vi "Wrist Controller.vi"(8 "error in":errorcluster) -> ()   [LabVIEW 2018]
doc: "This VI executes continuously carrying out the current operation and responding to updates or new operations. It will often contain the timing or control code that is difficult to place directly in TeleOp. This VI generally opens all sensors and motors and isolates the rest of the robot code from knowing how the operations are carried out."
uses:
  <vilib>/Rock Robotics/WPI/Framework/Completion Status.ctl
  Wrist Setpoints.ctl
  Wrist Operations.ctl
  <vilib>/Rock Robotics/WPI/MotorControl/WPI_MotorControlDeviceRef.ctl
  <vilib>/Rock Robotics/WPI/MotorControl/WPI_MotorControlType.ctl
  <vilib>/Rock Robotics/SystemInterfaces/DIO/FPGA_DIOPWMChannel.ctl
  <vilib>/Rock Robotics/WPI/PWM/WPI_PWMDeadband.ctl
  <vilib>/Rock Robotics/SystemInterfaces/DIO/FPGA_DIOChannel.ctl
  <vilib>/Rock Robotics/WPI/Counter/WPI_CounterDevRef.ctl
  <vilib>/Rock Robotics/SystemInterfaces/Counter/FPGA_CounterCtrSystemIndex.ctl
  <vilib>/Rock Robotics/WPI/ThirdParty/REV Robotics/SPARK MAX/Typedef/Spark MAX Control Type.ctl
  Wrist Published Globals.vi
panel:
  in  "Sensor Distance":dbl=190.0
  in  "0 Offset":dbl=160.0
  in  "Gravity Voltage":dbl=-0.5
  in  "upper limit":dbl=107.0
  in  "lower limit":dbl=-10.0
  in  "invert?":bool=TRUE
  in  "i Zone":dbl=inf format="%.2f"
  in  "PIDF gains":cluster{"Kp":dbl, "Ki":dbl, "Kd":dbl, "Kf":dbl}={"Kp"=0.03, "Ki"=0.0, "Kd"=0.0, "Kf"=0.0} {"Kf" format="%.3f"; "Kd" format="%.3f"; "Ki" format="%.3f"; "Kp" format="%.3f"}
  in  "output range":cluster{"output high":dbl, "output low":dbl}={"output high"=0.75, "output low"=-0.75} {"output low" format="%.2f"; "output high" format="%.2f"}
  out "Waveform Chart":T1(graph)={"output"=-0.11472656249999999, "upper limit"=105.0, "unwrapped phase"=101.17578125}
  in  "Interactive Values":T2={"Operation"=enum."Set Position", "Setpoint"=50.0, "Duration"=0.0}
  out "Current\nCmd":string="Started at  19:12:07.827\nDefault: Reserve,  S 0.0, D 0.000000"
  in  "Buttons":cluster{"Execute Cmd":bool, "Abort Cmd":bool}
  out "Command Timing":cluster{"Start Time (ms)":u32, "Iterations":i32}={"Start Time (ms)"=1785240, "Iterations"=0}
  out "Status":T4
  # "Interactive Command: You may fill in the settings for a command\nand schedule it with the Execute button. You can observe and abort\nany command while fine tuning the code for the controller."
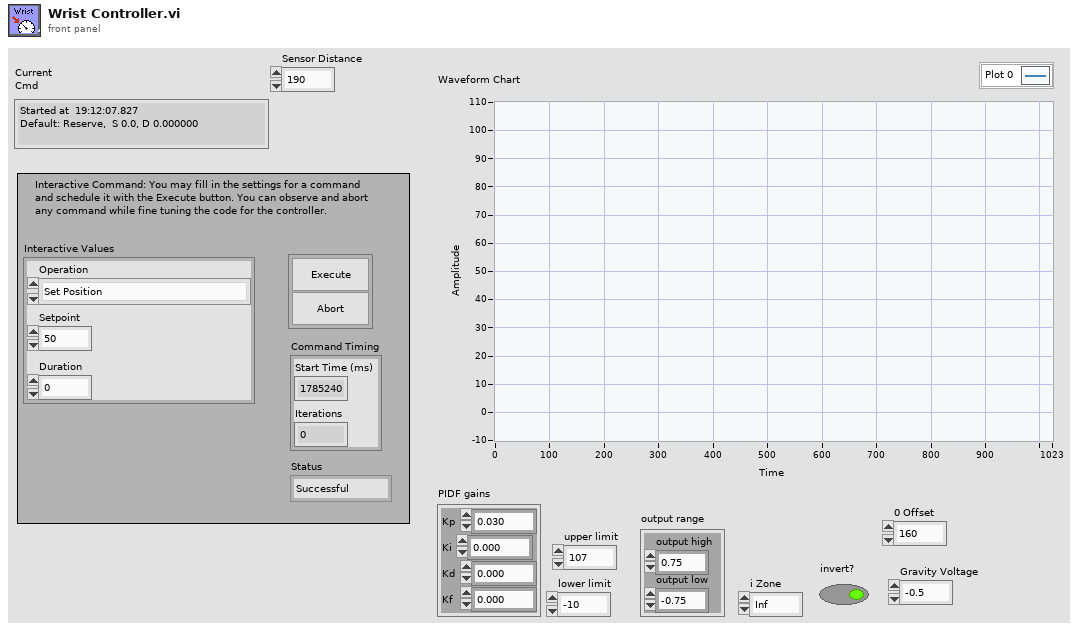
[diagram p1: front panel]
types:
  T1 = cluster{"output":dbl, "upper limit":dbl, "unwrapped phase":dbl}
  T2 = typedef "Wrist Setpoints.ctl" = cluster{"Operation":T3, "Setpoint":dbl, "Duration":dbl}
  T3 = typedef "Wrist Operations.ctl" = enum16{"Reserve", "Read Current", "Immediate", "Set Position"}
  T4 = typedef "Completion Status.ctl" = enum16{"Successful", "Aborted", "Incomplete"}
  T5 = typedef "WPI_MotorControlDeviceRef.ctl" = cluster{"DeviceStatus":errorcluster, "Type":T6, "PWM":cluster{"PWM Channel":T7, "DeadBand":T8}, "CAN":cluster{"Device Number":u8, "SetOutput VI Ref":variant, "GetOutput VI Ref":variant, "Enable VI Ref":variant, "Disable VI Ref":variant, "Data":variant}, "Invert":bool, "DIO PWM":cluster{"PWM \"Enable\" Channel":T7, "DIOChannel":T9, "PWM Rate":dbl}}
  T6 = typedef "WPI_MotorControlType.ctl" = enum16{"PWM", "CAN", "DIO PWM"}
  T7 = typedef "FPGA_DIOPWMChannel.ctl" = enum8{"PWM 0", "PWM 1", "PWM 2", "PWM 3", "PWM 4", "PWM 5", "PWM 6", "PWM 7", "PWM 8", "PWM 9", "PWM MXP 0", "PWM MXP 1", "PWM MXP 2", "PWM MXP 3", "PWM MXP 4", "PWM MXP 5", "PWM MXP 6", "PWM MXP 7", "PWM MXP 8", "PWM MXP 9", "Invalid"}
  T8 = typedef "WPI_PWMDeadband.ctl" = cluster{"Name":string, "maxPositivePwm":i32, "minPositivePwm":i32, "centerPwm":i32, "maxNegativePwm":i32, "minNegativePwm":i32, "angularRange":u16}
  T9 = typedef "FPGA_DIOChannel.ctl" = enum8{"DIO 0", "DIO 1", "DIO 2", "DIO 3", "DIO 4", "DIO 5", "DIO 6", "DIO 7", "DIO 8", "DIO 9", "DIO MXP 0", "DIO MXP 1", "DIO MXP 2", "DIO MXP 3", "DIO MXP 4", "DIO MXP 5", "DIO MXP 6", "DIO MXP 7", "DIO MXP 8", "DIO MXP 9", "DIO MXP 10", "DIO MXP 11", "DIO MXP 12", "DIO MXP 13", "DIO MXP 14", "DIO MXP 15", "SPI Port CS1", "SPI Port CS2", "SPI Port CS3", "SPI Port MISO", "SPI Port MOSI", "Invalid"}
  T10 = typedef "WPI_CounterDevRef.ctl" = cluster{"DevStatus":errorcluster, "CntIndex":T11}
  T11 = typedef "FPGA_CounterCtrSystemIndex.ctl" = enum8{"Ctr 0", "Ctr 1", "Ctr 2", "Ctr 3", "Ctr 4", "Ctr 5", "Ctr 6", "Ctr 7", "Invalid"}
  T12 = cluster{"Motor":T5, "Sensor":T10, "Setpoint":dbl, "Cargo Detect":T10}
  T13 = typedef "Command Status Info.ctl" = cluster{"Name":string, "Status":T4, "notifier out":T14}
  T14 = typedef "Completion Notifier.ctl" = refnum<notifier>
  T15 = cluster{"Current Command":T2, "Command Timing":cluster{"Start Time (ms)":u32, "Iterations":i32}, "Command Arguments":cluster{"Command Info":T13, "Description":string, "Default Command":T2, "queue out":refnum<queue>, "Subsystem Name":string}}
  T16 = typedef "Spark MAX Control Type.ctl" = enum16{"Percent VBus", "Voltage", "Velocity", "Position", "Smart Motion", "Current", "Smart Velocity"}
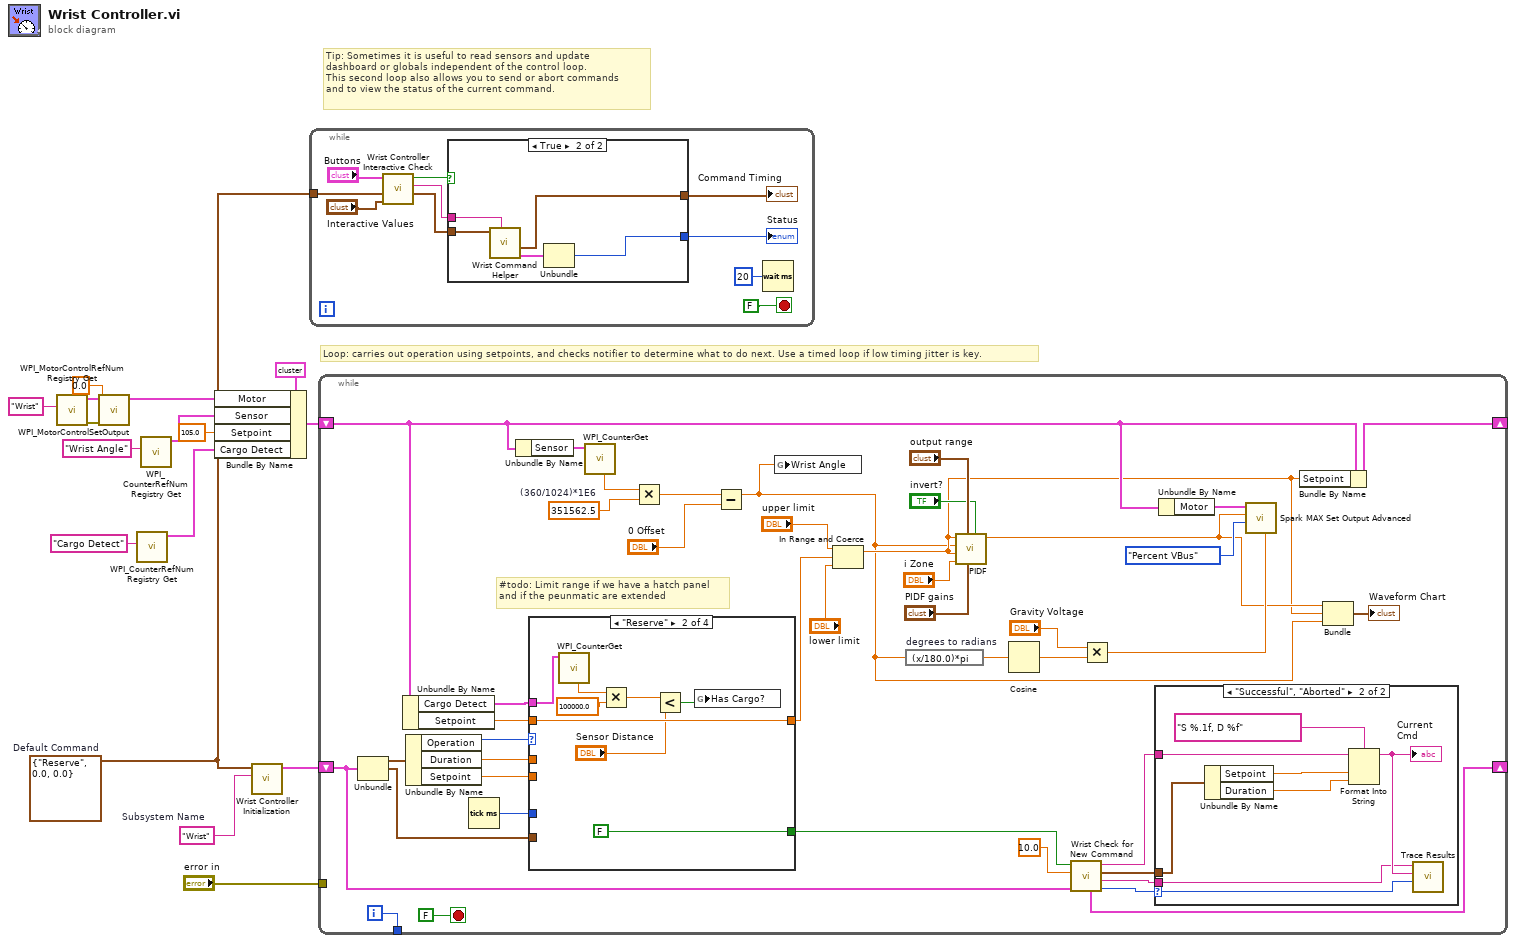
[diagram p0: block diagram]
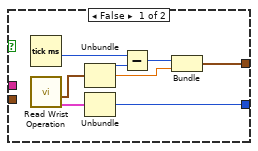
[diagram p2: hidden frame]
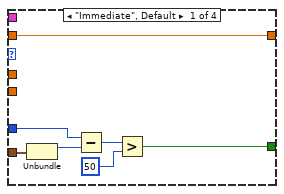
[diagram p4: hidden frame]
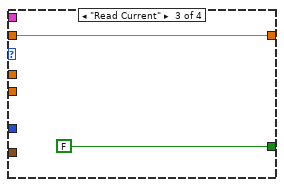
[diagram p5: hidden frame]
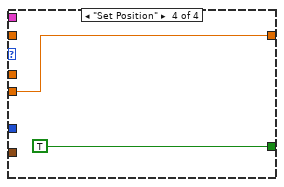
[diagram p6: hidden frame]
diagram:
  w13 = T2 {"Operation"=enum."Reserve", "Setpoint"=0.0, "Duration"=0.0}  # Default Command
  w14 = "Wrist"  # Subsystem Name
  # "Tip: Sometimes it is useful to read sensors and update\ndashboard or globals independent of the control loop.\nThis second loop also allows you to send or abort commands\nand to view the status of the current command."
  # "Loop: carries out operation using setpoints, and checks notifier to determine what to do next. Use a timed loop if low timing jitter is key."
  n1 = call <vilib>:"WPI_MotorControlRefNum Registry Get.vi"("refnum name"="Wrist") -> ("error out"=w5:errorcluster, "MotorControlDevRef"=w6:T5)  [unwired: 9 in]
  n2 = call <vilib>:"WPI_MotorControlSetOutput.vi"("error in (no error)"=w5, "Output"=0.0, "MotorControlDevRef"=w6) -> ("MotorControlDevRef"=w4:T5)  [unwired: 6 in, 2 out]
  n3 = call <vilib>:"WPI_CounterRefNum Registry Get.vi"("refnum name"="Cargo Detect") -> ("CounterDevRef"=w1:T10)  [unwired: 9 in, 1 out]
  n4 = call <vilib>:"WPI_CounterRefNum Registry Get.vi"("refnum name"="Wrist Angle") -> ("CounterDevRef"=w8:T10)  [unwired: 9 in, 1 out]
  n5 = Bundle By Name(cluster=T12 {"Motor"={"DeviceStatus"={"status"=FALSE, "code"=0, "source"=""}, "Type"=enum."PWM", "PWM"={"PWM Channel"=enum."Invalid", "DeadBand"={"Name"="", "maxPositivePwm"=0, "minPositivePwm"=0, "centerPwm"=0, "maxNegativePwm"=0, "minNegativePwm"=0, "angularRange"=0}}, "CAN"={"Device Number"=0, "SetOutput VI Ref"=variant(refnum<vi> refnum), "GetOutput VI Ref"=variant(refnum<vi> refnum), "Enable VI Ref"=variant(refnum<vi> refnum), "Disable VI Ref"=variant(refnum<vi> refnum), "Data"=variant}, "Invert"=FALSE, "DIO PWM"={"PWM \"Enable\" Channel"=enum."Invalid", "DIOChannel"=enum."Invalid", "PWM Rate"=0.0}}, "Sensor"={"DevStatus"={"status"=FALSE, "code"=0, "source"=""}, "CntIndex"=enum."Ctr 0"}, "Setpoint"=0.0, "Cargo Detect"={"DevStatus"={"status"=FALSE, "code"=0, "source"=""}, "CntIndex"=enum."Ctr 0"}}, "Motor"=w4, "Sensor"=w8, "Setpoint"=105.0, "Cargo Detect"=w1) -> (w9:T12)
  n6 = call "Wrist Controller Initialization.vi"("Subsystem Name"=w14, "Default Command"=w13) -> ("Current Command"=w15:T15)  [unwired: 9 in]
  n7 = while {
    tunnel: w13 -> [w23]
    stop <- FALSE stop-if-true
    n8 = call "Wrist Controller Interactive Check.vi"("Interactive Command in"="Interactive Values", "Default Command"=w23, "Buttons"="Buttons") -> ("Interactive Command out"=w20:T2, "Trace String"=w21:string, "Schedule"=w22:bool)  [unwired: 6 in]
    n9 = case shown="True" w22 {
      tunnel: [w34 w39] -> w19
      tunnel: w20 -> [_ w37]
      tunnel: [w30 w35] -> w18
      tunnel: w21 -> [_ w38]
      frame False {
        n10 = Tick Count (ms)() -> (millisecond timer value=w29:u32)
        n11 = call "Read Wrist Operation.vi"() -> ("Command Info"=w27:T13, "SubSystem Data"=w28:T2)  [unwired: 9 in, 1 out]
        n12 = Unbundle(w28) -> ("Operation"=w33:T3, "Setpoint"=w31:dbl)  [unwired: 1 out]
        n13 = Unbundle(w27) -> ("Status"=w34:T4)  [unwired: 2 out]
        n14 = Subtract(x=w29, y=w33) -> (x-y=w32:u32)
        n15 = Bundle(w32, "Setpoint"=w31) -> (w30:cluster{u32, "Setpoint":dbl})  [unwired: 1 in]
      }
      frame True {
        n16 = call "Wrist Command Helper.vi"("Description"=w38, "SubSystem Data"=w37) -> ("Command Info Out"=w36:T13, "Command Timing"=w35:cluster{"Start Time (ms)":u32, "Iterations":i32})  [unwired: 7 in, 1 out]
        n17 = Unbundle(w36) -> ("Status"=w39:T4)  [unwired: 2 out]
      }
    }
    "Status" <- w19
    "Command Timing" <- w18
    n18 = Wait (ms)(milliseconds to wait=u32 20) -> ()  [unwired: 1 out]
  }
  n19 = while {
    shift-right: [w73] -> _
    shift-left: w15 -> [w67]
    tunnel: [w80] -> _
    tunnel: "error in" -> [_]
    shift-right: [w58] -> _
    shift-left: w9 -> [w56]
    i -> [w80]
    stop <- FALSE stop-if-true
    w63 = 351562.5  # (360/1024)*1E6
    # "#todo: Limit range if we have a hatch panel\nand if the peunmatic are extended"
    n20 = Unbundle(w67) -> ("Current Command"=w79:T2, "Command Timing"=w75:cluster{"Start Time (ms)":u32, "Iterations":i32})  [unwired: 1 out]
    n21 = Unbundle By Name(w56) -> ("Cargo Detect"=w40:T10, "Setpoint"=w59:dbl)
    n22 = Unbundle By Name(w79) -> ("Operation"=w78:T3, "Duration"=w77:dbl, "Setpoint"=w74:dbl)
    n23 = Tick Count (ms)() -> (millisecond timer value=w76:u32)
    n24 = Unbundle By Name(w56) -> ("Sensor"=w65:T10)
    n25 = case shown="\"Reserve\"" w78 {
      tunnel: [w91 FALSE ("ignore previous (F)") FALSE ("ignore previous (F)") TRUE ("ignore previous (F)")] -> w72
      tunnel: w75 -> [w93 _ _ _]
      tunnel: w77 -> [_ _ _ _]
      tunnel: w76 -> [w92 _ _ _]
      tunnel: w74 -> [_ _ _ w107]
      tunnel: w59 -> [w90 w103 w105 _]
      tunnel: [w90 w103 w105 w107] -> w55
      tunnel: w40 -> [_ w102 _ _]
      frame "Immediate", Default {
        n26 = Unbundle(w93) -> ("Start Time (ms)"=w96:u32)  [unwired: 1 out]
        n27 = Subtract(x=w92, y=w96) -> (x-y=w95:u32)
        n28 = Greater?(x=w95, y=u8 50 ("Left Motor")) -> (0:w91:bool)
      }
      frame "Reserve" {
        n29 = call <vilib>:"WPI_CounterGet.vi"("CounterDevRef in"=w102) -> ("Period (sec)"=w101:dbl)  [unwired: 5 in, 5 out]
        n30 = Multiply(x=w101, y=100000.0) -> (x*y=w99:dbl)
        n31 = Less?(x=w99, y="Sensor Distance") -> (x < y?=w97:bool)
        n32 = global write "Wrist Published Globals.vi" "Has Cargo?"(w97) -> ()
      }
      frame "Read Current" {
      }
      frame "Set Position" {
      }
    }
    n33 = call <vilib>:"WPI_CounterGet.vi"("CounterDevRef in"=w65) -> ("Period (sec)"=w64:dbl)  [unwired: 5 in, 5 out]
    n34 = Multiply(x=w64, y=w63) -> (x*y=w43:dbl)
    n35 = Subtract(x=w43, y="0 Offset") -> (x-y=w41:dbl)
    n36 = global write "Wrist Published Globals.vi" "Wrist Angle"(w41) -> ()
    n37 = In Range and Coerce(upper limit="upper limit", x=w55, lower limit="lower limit") -> (coerced(x)=w45:dbl)  [unwired: 1 out]
    n38 = expression code="(x/180.0)*pi" "degrees to radians"(w41) -> (w50:dbl)
    n39 = call "PIDF.vi"("invert? (F)"="invert?", "PIDF gains"="PIDF gains", "output range"="output range", "i Zone"="i Zone", "Feedforward"=w45, "process variable"=w41, "setpoint"=w45) -> ("output"=w46:dbl)  [unwired: 2 in, 2 out]
    n40 = Cosine(x=w50) -> (cos(x)=w49:dbl)
    n41 = call "Wrist Check for New Command.vi"("Current Command"=w67, "Wait time (ms)"=10.0, "Finished?"=w72) -> ("Completion"=w68:T4, "Subsystem Name"=w69:string, "Current Command"=w70:T2, "Initial Trace String"=w71:string, "NextCommand"=w73:T15)  [unwired: 4 in]
    n42 = Multiply(x="Gravity Voltage", y=w49) -> (x*y=w47:dbl)
    n43 = case shown="\"Successful\", \"Aborted\"" w68 {
      selector: w68 -> [_ w89]
      tunnel: w71 -> [_ w85]
      tunnel: w70 -> [_ w86]
      tunnel: w69 -> [_ w82]
      frame "Incomplete", Default {
        # "Continuing current command"
      }
      frame "Successful", "Aborted" {
        # "Report and setup for next command"
        n44 = Unbundle By Name(w86) -> ("Setpoint"=w88:dbl, "Duration"=w83:dbl)
        n45 = Format Into String(format string="S %.1f, D %f", initial string=w85, w88, w83) -> (resulting string=w84:string)  [unwired: 1 in, 1 out]
        "Current\nCmd" <- w84
        n46 = call <vilib>:"Trace Results.vi"("Status of previous command"=w89, "Description"=w84, "Subsystem"=w82) -> ()  [unwired: 9 in]
      }
    }
    n47 = Unbundle By Name(w56) -> ("Motor"=w52:T5)
    n48 = call <vilib>:"Spark MAX Set Output Advanced.vi"("Arbitrary Feed Forward (0)"=w47, "Control Mode"=Spark_MAX_Control_Type."Percent VBus", "Setpoint"=w46, "MotorControlDevRef"=w52) -> ()  [unwired: 6 in, 2 out]
    n49 = Bundle By Name(cluster=w56, "Setpoint"=w45) -> (w58:T12)
    n50 = Bundle("output"=w46, "upper limit"=w45, w41) -> (→"Waveform Chart":cluster{"output":dbl, "upper limit":dbl, dbl})  [unwired: 1 in]
  }
